vi "Test - Replace Row Or Column.vi"() -> ()   [LabVIEW 2022 SP3, in "Raster.lvlib"]
uses:
  Raster.lvlib
  <vilib>/Utility/High Resolution Relative Seconds.vi
  Utility/Utility.lvlib
panel:
  out "Array 2":dbl[][](array[numeric])
  out "Array":dbl[][](array[numeric])
  out "Delta Time [s] 2":dbl format="%.3p"
  out "Delta Time [s]":dbl format="%.3p"
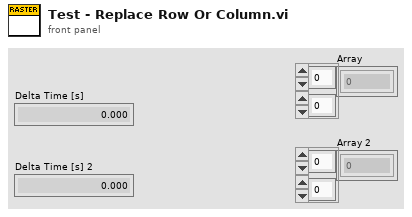
[diagram p1: front panel]
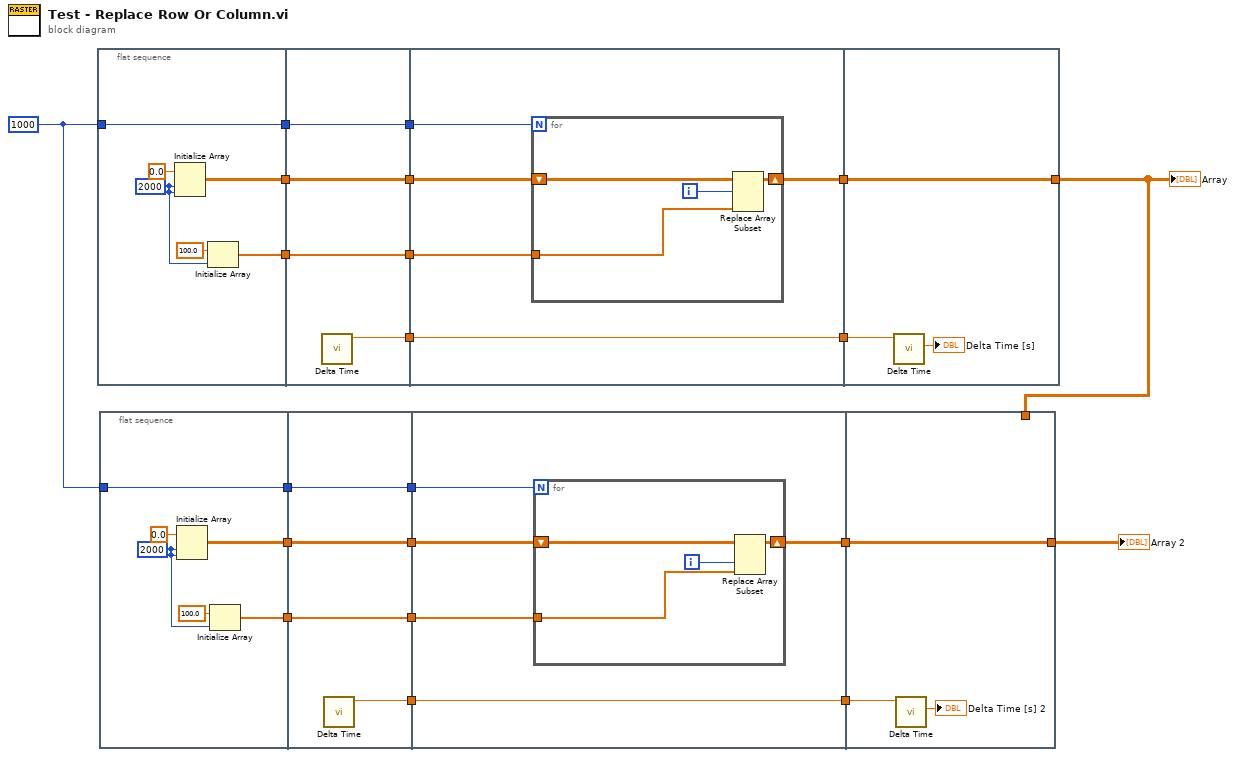
[diagram p0: block diagram]
diagram:
  w3 = 1000
  n1 = flat-sequence {
    tunnel: [w26] -> w19
    tunnel: [w23] -> w17
    tunnel: [w22] -> w6
    tunnel: w3 -> [w22]
    tunnel: w19 -> [w31]
    tunnel: [w31] -> w18
    tunnel: w17 -> [w30]
    tunnel: [w30] -> w16
    tunnel: [w29] -> w15
    tunnel: [w28] -> w7
    tunnel: w6 -> [w28]
    tunnel: w18 -> [w36]
    tunnel: w16 -> [w35]
    tunnel: w15 -> [w34]
    tunnel: [w34] -> w21
    tunnel: [w33] -> w20
    tunnel: w7 -> [w32]
    tunnel: w21 -> [w43]
    tunnel: w20 -> [w41]
    tunnel: [w41] -> w1
    frame #0 {
      w24 = 2000 ("dimension size")
      n2 = Initialize Array(0.0 ("element"), w24, w24) -> (w26:dbl[][])
      n3 = Initialize Array(100.0 ("element"), w24) -> (w23:dbl[])
    }
    frame #1 {
      n4 = call "Delta Time.vi"() -> ("Relative Seconds Out"=w29:dbl)  [unwired: 10 in, 1 out]
    }
    frame #2 {
      n5 = for {
        N: w32 -> [_]
        shift-right: [w38] -> w33
        shift-left: w36 -> [w40]
        tunnel: w35 -> [w39]
        i -> [w37]
        n6 = Replace Array Subset(array=w40, new element=w39, index (row)=w37) -> (w38:dbl[][])  [unwired: 1 in]
      }
    }
    frame #3 {
      n7 = call "Delta Time.vi"("Relative Seconds In"=w43) -> ("Delta Time [s]"=→"Delta Time [s]":dbl)  [unwired: 9 in, 1 out]
    }
  }
  n8 = flat-sequence {
    tunnel: [w48] -> w14
    tunnel: [w45] -> w13
    tunnel: [w44] -> w4
    tunnel: w3 -> [w44]
    tunnel: w14 -> [w53]
    tunnel: [w53] -> w12
    tunnel: w13 -> [w52]
    tunnel: [w52] -> w11
    tunnel: [w51] -> w10
    tunnel: [w50] -> w5
    tunnel: w4 -> [w50]
    tunnel: w12 -> [w58]
    tunnel: w11 -> [w57]
    tunnel: w10 -> [w56]
    tunnel: [w56] -> w9
    tunnel: [w55] -> w8
    tunnel: w5 -> [w54]
    tunnel: w9 -> [w65]
    tunnel: w8 -> [w63]
    tunnel: [w63] -> w2
    tunnel: w1 -> [_]
    frame #0 {
      w46 = 2000 ("dimension size")
      n9 = Initialize Array(0.0 ("element"), w46, w46) -> (w48:dbl[][])
      n10 = Initialize Array(100.0 ("element"), w46) -> (w45:dbl[])
    }
    frame #1 {
      n11 = call "Delta Time.vi"() -> ("Relative Seconds Out"=w51:dbl)  [unwired: 10 in, 1 out]
    }
    frame #2 {
      n12 = for {
        N: w54 -> [_]
        shift-right: [w60] -> w55
        shift-left: w58 -> [w62]
        tunnel: w57 -> [w61]
        i -> [w59]
        n13 = Replace Array Subset(array=w62, new element=w61, index (col)=w59) -> (w60:dbl[][])  [unwired: 1 in]
      }
    }
    frame #3 {
      n14 = call "Delta Time.vi"("Relative Seconds In"=w65) -> ("Delta Time [s]"=→"Delta Time [s] 2":dbl)  [unwired: 9 in, 1 out]
    }
  }
  "Array" <- w1
  "Array 2" <- w2
